vi "fgv_ROI equal size line coords.vi"(8 "error in (no error)":errorcluster, 9 "New Line Coordinates":i32[](array[numeric]), 11 "Function":enum16{"Intialize", "Write", "Read", "Clear"}(ring)) -> (0 "error out":errorcluster, 1 "Registered Line Coordinates":i32[](array[numeric]))   [LabVIEW 2020]
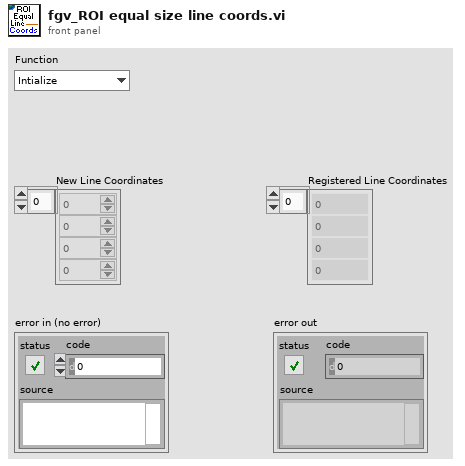
[diagram p1: front panel]
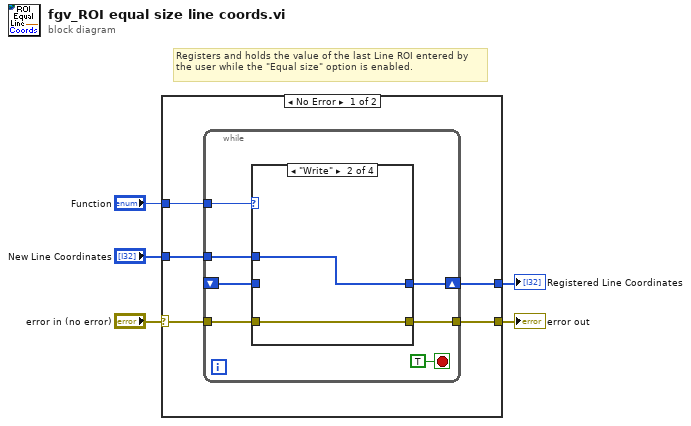
[diagram p0: block diagram]
diagram:
  # "Registers and holds the value of the last Line ROI entered by the user while the \"Equal size\" option is enabled."
  n1 = case shown="No Error" "error in (no error)" {
    selector: "error in (no error)" -> [w8 w25]
    tunnel: [w9 w25] -> w4
    tunnel: "Function" -> [w10 _]
    tunnel: "New Line Coordinates" -> [w7 w24]
    tunnel: [w6 w24] -> w1
    frame No Error {
      n2 = while {
        tunnel: w10 -> [w16]
        tunnel: [w14] -> w9
        tunnel: w8 -> [w15]
        tunnel: w7 -> [w13]
        shift-right: [w12] -> w6
        shift-left: _ -> [w11]
        stop <- TRUE stop-if-true
        n3 = case shown="\"Write\"" w16 {
          tunnel: [w18 w20 w22 w23] -> w14
          tunnel: w15 -> [w18 w20 w22 w23]
          tunnel: w13 -> [_ w19 _ _]
          tunnel: [_ w19 w21 _] -> w12
          tunnel: w11 -> [_ _ w21 _]
          frame "Intialize", Default {
          }
          frame "Write" {
          }
          frame "Read" {
          }
          frame "Clear" {
          }
        }
      }
    }
    frame Error {
    }
  }
  "error out" <- w4
  "Registered Line Coordinates" <- w1
